vi "uc480_SubVI_Example_GetFramerate.vi"(0 ".NET (Reference)":refnum<k24>, 11 "Error In":errorcluster) -> (4 "Framerate":dbl, 6 "Inc":dbl, 8 "Min":dbl, 10 "Max":dbl, 15 "error out":errorcluster caption="Error Out")   [LabVIEW 2015]
uses:
  C:/Program Files/Thorlabs/Scientific Imaging/DCx Camera Support/Develop/DotNet/uc480DotNet.dll
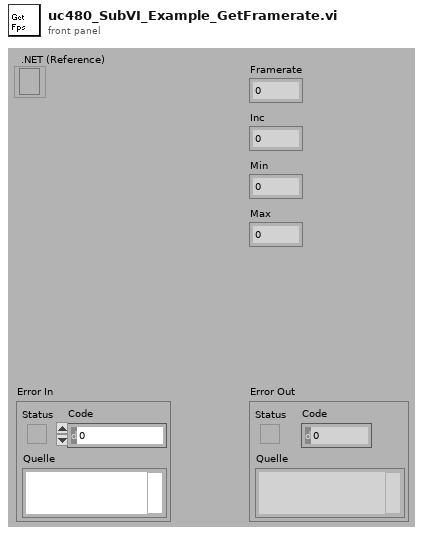
[diagram p1: front panel]
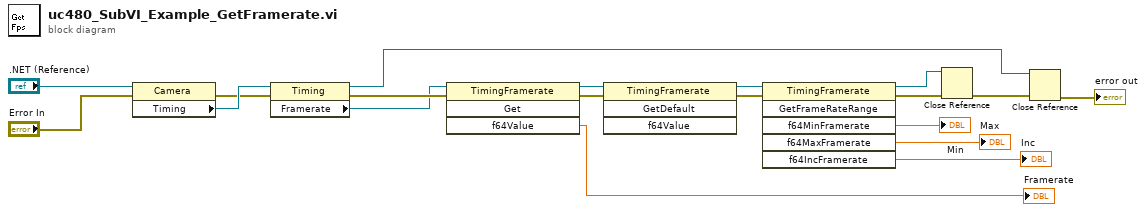
[diagram p0: block diagram]
diagram:
  n1 = property class="Camera"(reference=".NET (Reference)", error in="Error In") -> (error out=w18:errorcluster, "Timing"=w19:refnum<k24>)  [unwired: 1 out]
  n2 = property class="Timing"(reference=w19, error in=w18) -> (reference out=w3:refnum<k24>, error out=w17:errorcluster, "Framerate"=w16:refnum<k24>)
  n3 = invoke class="TimingFramerate" method="Get"(reference=w16, error in=w17) -> (reference out=w15:refnum<k24>, error out=w14:errorcluster, "f64Value"=→"Framerate":dbl)  [unwired: 2 in, 1 out]
  n4 = invoke class="TimingFramerate" method="GetDefault"(reference=w15, error in=w14) -> (reference out=w12:refnum<k24>, error out=w13:errorcluster)  [unwired: 2 in, 2 out]
  n5 = invoke class="TimingFramerate" method="GetFrameRateRange"(reference=w12, error in=w13) -> (reference out=w4:refnum<k24>, error out=w5:errorcluster, "f64MinFramerate"=→"Min":dbl, "f64MaxFramerate"=→"Max":dbl, "f64IncFramerate"=→"Inc":dbl)  [unwired: 4 in, 1 out]
  n6 = Close Reference(reference=w4, error in (no error)=w5) -> (error out=w2:errorcluster)
  n7 = Close Reference(reference=w3, error in (no error)=w2) -> (error out=→"error out":errorcluster)
